vi "delete.vi"(8 "error in (no error)":errorcluster, 10 "current node":refnum<class "Iterator.lvclass">, 11 "DoublyLinkedList in":refnum<class "DoublyLinkedList.lvclass">) -> (0 "error out":errorcluster, 3 "DoublyLinkedList out":refnum<class "DoublyLinkedList.lvclass">)   [LabVIEW 2021, in "DoublyLinkedList.lvclass"]
uses:
  DoublyLinkedList.lvclass
  Iterator/Iterator.lvclass
  DoublyLinkedList.lvclass/DoublyLinkedList.ctl
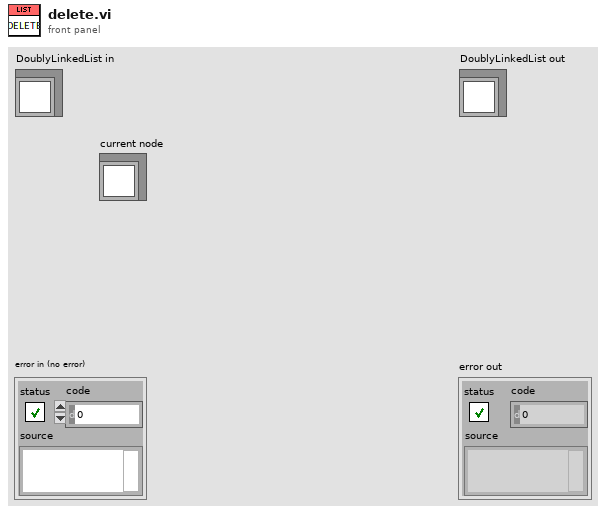
[diagram p1: front panel]
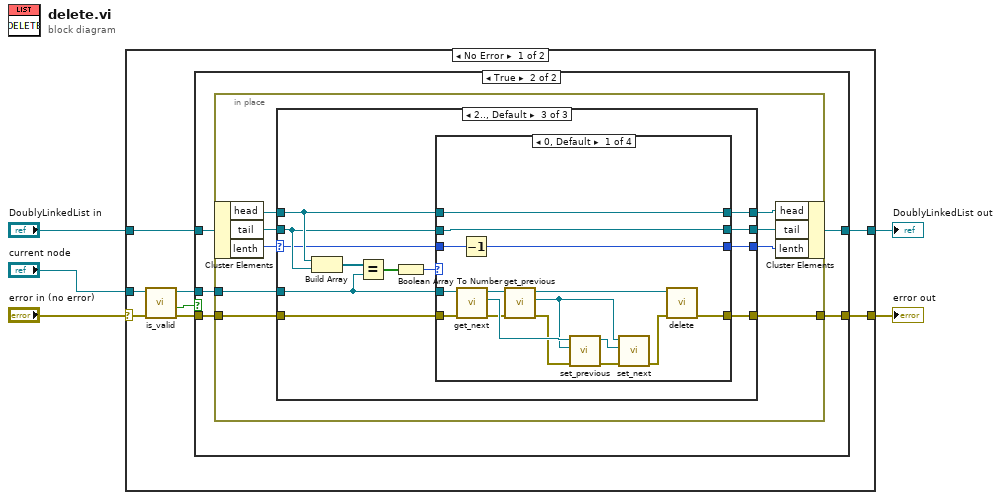
[diagram p0: block diagram]
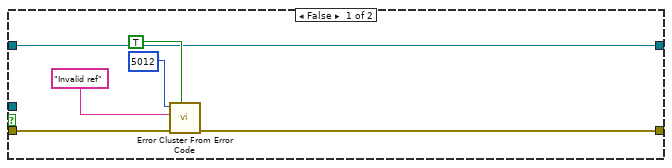
[diagram p2: hidden frame]
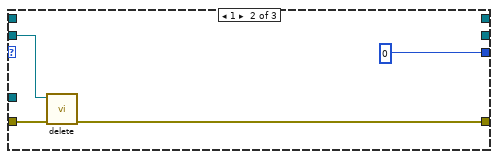
[diagram p4: hidden frame]
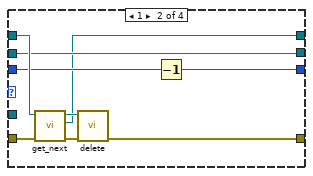
[diagram p5: hidden frame]
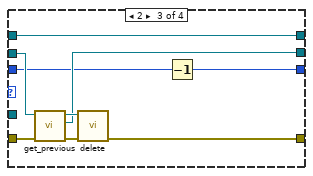
[diagram p6: hidden frame]
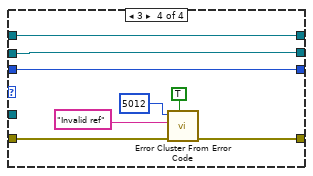
[diagram p7: hidden frame]
diagram:
  n1 = case shown="No Error" "error in (no error)" {
    selector: "error in (no error)" -> [w9 w97]
    tunnel: [w12 w97] -> w1
    tunnel: [w11 w96] -> w2
    tunnel: "DoublyLinkedList in" -> [w13 w96]
    tunnel: "current node" -> [w10 _]
    frame No Error {
      n2 = call-dynamic "is_valid.vi"("error in (no error)"=w9, "Iterator in"=w10) -> ("error out"=w8:errorcluster, "valid?"=w7:bool, "Iterator out"=w6:refnum<class "Iterator.lvclass">)  [unwired: 7 in]
      n3 = case shown="True" w7 {
        tunnel: w13 -> [w14 w24]
        tunnel: w8 -> [w16 w23]
        tunnel: [w15 w22] -> w12
        tunnel: [w14 w21] -> w11
        tunnel: w6 -> [_ w20]
        frame False {
          n4 = call <vilib>:"Error Cluster From Error Code.vi"("show call chain? (False)"=TRUE, "error in (no error)"=w16, "error message (\"\")"="Invalid ref" ("error message (\"\")"), "error code (0)"=5012) -> ("error out"=w15:errorcluster)  [unwired: 5 in]
        }
        frame True {
          n5 = in-place {
            in-place-border: w23 -> [w26]
            in-place-border: [w29] -> w22
            in-place-border: w20 -> [w25]
            n6 = in-place-cluster #1(w24) -> ("head"=w33:refnum<class "Iterator.lvclass">, "tail"=w32:refnum<class "Iterator.lvclass">, "lenth"=w28:u32)
            n7 = case shown="2.., Default" w28 {
              selector: w28 -> [w37 _ w44]
              tunnel: [w35 _ w45] -> w30
              tunnel: w33 -> [w34 _ w51]
              tunnel: w32 -> [w35 w40 w46]
              tunnel: [w34 _ w53] -> w31
              tunnel: [w36 w38 w52] -> w29
              tunnel: [w37 u32 0 ("lenth") w43] -> w27
              tunnel: w26 -> [w36 w39 w47]
              tunnel: w25 -> [_ _ w42]
              frame 0 {
              }
              frame 1 {
                n8 = call-dynamic "delete.vi"("error in (no error)"=w39, "Iterator in"=w40) -> ("error out"=w38:errorcluster)  [unwired: 9 in]
              }
              frame 2.., Default {
                n9 = Build Array(w51, w46) -> (w50:refnum<class "Iterator.lvclass">[])
                n10 = Equal?(x=w50, y=w42) -> (x = y?=w49:bool[])
                n11 = Boolean Array To Number(Boolean array=w49) -> (number=w48:u32)
                n12 = case shown="0, Default" w48 {
                  tunnel: [w67 w70 w85 w90] -> w53
                  tunnel: [w54 w71 w81 w91] -> w52
                  tunnel: w51 -> [w67 w76 w85 w90]
                  tunnel: w47 -> [w60 w72 w83 w92]
                  tunnel: w46 -> [w68 w74 w84 w89]
                  tunnel: [w68 w74 w82 w89] -> w45
                  tunnel: w44 -> [w66 w75 w80 w88]
                  tunnel: [w65 w73 w79 w88] -> w43
                  tunnel: w42 -> [w69 _ _ _]
                  frame 0, Default {
                    n13 = call-dynamic "get_next.vi"("error in (no error)"=w60, "Iterator in"=w69) -> ("error out"=w59:errorcluster, "next"=w63:refnum<class "Iterator.lvclass">, "Iterator out"=w64:refnum<class "Iterator.lvclass">)  [unwired: 6 in, 1 out]
                    n14 = Decrement(x=w66) -> (x-1=w65:u32)
                    n15 = call-dynamic "get_previous.vi"("error in (no error)"=w59, "Iterator in"=w64) -> ("error out"=w58:errorcluster, "previous"=w62:refnum<class "Iterator.lvclass">, "Iterator out"=w56:refnum<class "Iterator.lvclass">)  [unwired: 6 in, 1 out]
                    n16 = call-dynamic "set_previous.vi"("error in (no error)"=w58, "previous"=w62, "Iterator in"=w63) -> ("error out"=w57:errorcluster, "Iterator out"=w61:refnum<class "Iterator.lvclass">)  [unwired: 7 in]
                    n17 = call-dynamic "set_next.vi"("error in (no error)"=w57, "next"=w61, "Iterator in"=w62) -> ("error out"=w55:errorcluster)  [unwired: 7 in, 1 out]
                    n18 = call-dynamic "delete.vi"("error in (no error)"=w55, "Iterator in"=w56) -> ("error out"=w54:errorcluster)  [unwired: 9 in]
                  }
                  frame 1 {
                    n19 = call-dynamic "get_next.vi"("error in (no error)"=w72, "Iterator in"=w76) -> ("error out"=w78:errorcluster, "next"=w70:refnum<class "Iterator.lvclass">, "Iterator out"=w77:refnum<class "Iterator.lvclass">)  [unwired: 6 in, 1 out]
                    n20 = call-dynamic "delete.vi"("error in (no error)"=w78, "Iterator in"=w77) -> ("error out"=w71:errorcluster)  [unwired: 9 in]
                    n21 = Decrement(x=w75) -> (x-1=w73:u32)
                  }
                  frame 2 {
                    n22 = call-dynamic "get_previous.vi"("error in (no error)"=w83, "Iterator in"=w84) -> ("error out"=w87:errorcluster, "previous"=w82:refnum<class "Iterator.lvclass">, "Iterator out"=w86:refnum<class "Iterator.lvclass">)  [unwired: 6 in, 1 out]
                    n23 = call-dynamic "delete.vi"("error in (no error)"=w87, "Iterator in"=w86) -> ("error out"=w81:errorcluster)  [unwired: 9 in]
                    n24 = Decrement(x=w80) -> (x-1=w79:u32)
                  }
                  frame 3 {
                    n25 = call <vilib>:"Error Cluster From Error Code.vi"("show call chain? (False)"=TRUE, "error in (no error)"=w92, "error message (\"\")"="Invalid ref" ("error message (\"\")"), "error code (0)"=5012) -> ("error out"=w91:errorcluster)  [unwired: 5 in]
                  }
                }
              }
            }
            n26 = in-place-cluster #1("head"=w31, "tail"=w30, "lenth"=w27) -> (w21:refnum<class "DoublyLinkedList.lvclass">)
          }
        }
      }
    }
    frame Error {
    }
  }
  "error out" <- w1
  "DoublyLinkedList out" <- w2
